vi "Get Available Data Channels.vi"(8 "error in (no error)":errorcluster, 10 "MetaData":refnum<vi>, 11 "Item Ref in":T1 format="%.0x") -> (0 "error out":errorcluster, 3 "Item Ref out":T1 format="%.0x")   [LabVIEW 2019, in "Instrument Addon System Explorer.lvlib"]
uses:
  Instrument Addon System Explorer.lvlib
  <vilib>/NI VeriStand/Custom Device API/Custom Device API.lvlib
  <vilib>/NI VeriStand/Custom Device API/Get Item Property (String).vi
  Shared/Constants.vi
  Shared/Instrument Addon Shared.lvlib
  <vilib>/NI VeriStand/Custom Device API/Custom Device Item Ref.ctl
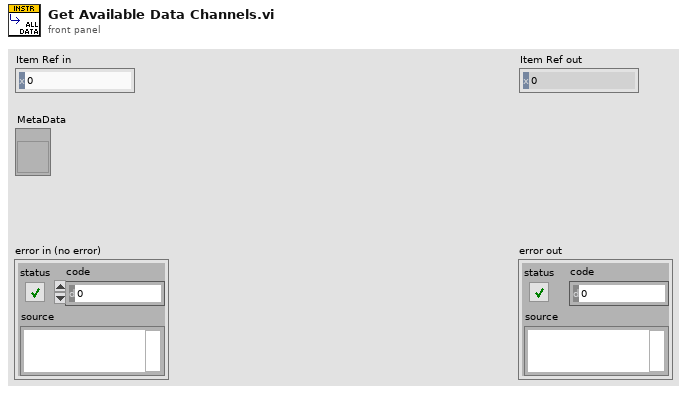
[diagram p1: front panel]
types:
  T1 = typedef "Custom Device API.lvlib/Custom Device Item Ref.ctl" = u64
  T2 = typedef "Custom Device API.lvlib/Custom Device Item Info.ctl" = cluster{"Name":string, "Is Channel":bool, "GUID":string, "Is Waveform":bool}
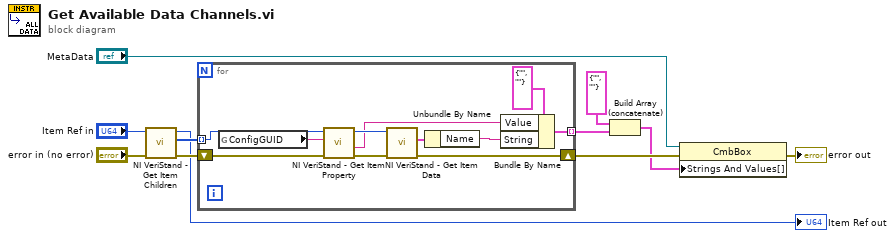
[diagram p0: block diagram]
diagram:
  n1 = call <vilib>:"NI VeriStand - Get Item Children.vi"("error in (no error)"="error in (no error)", "Item Ref in"="Item Ref in") -> ("error out"=w10:errorcluster, "Child Refs"=w11:T1[], "Item Ref out"=→"Item Ref out":T1)  [unwired: 6 in, 1 out]
  n2 = for {
    tunnel: w11 -> [w13] mode=indexing
    shift-right: [w21] -> w9
    shift-left: w10 -> [w16]
    tunnel: [w19] -> w7 mode=indexing
    n3 = global read "Constants.vi" "ConfigGUID"() -> (w17:string)
    n4 = call-poly <vilib>:"NI VeriStand - Get Item Property.vi"("error in (no error)"=w16, "Property Name"=w17, "Item Ref in"=w13) -> ("error out"=w15:errorcluster, "Value"=w12:string, "Item Ref out"=w14:T1)  [unwired: 5 in, 1 out]
    n5 = call <vilib>:"NI VeriStand - Get Item Data.vi"("error in (no error)"=w15, "Item Ref in"=w14) -> ("error out"=w21:errorcluster, "Item Info"=w22:T2)  [unwired: 8 out]
    n6 = Unbundle By Name(w22) -> ("Name"=w20:string)
    n7 = Bundle By Name(cluster=cluster{"String":string, "Value":string} {"String"="", "Value"=""}, "Value"=w12, "String"=w20) -> (w19:cluster{"String":string, "Value":string})
  }
  n8 = Build Array (concatenate)(cluster{"String":string, "Value":string} {"String"="", "Value"=""}, w7) -> (w1:cluster{"String":string, "Value":string}[])
  n9 = property class="CmbBox"(reference="MetaData", error in=w9, "Strings And Values[]"=w1) -> (error out=→"error out":errorcluster)  [unwired: 1 out]
